vi "Weird Master.vi"() -> ()   [LabVIEW 2021]
uses:
  Transmission Data Unit/RTU/RTU Data Unit.lvclass
  API/Master/Modbus Master.lvclass
  Transmission Data Unit/ASCII/ASCII Data Unit.lvclass
  Network Protocol/Network Master/TCP/TCP Master.lvclass
  Master Function Definition/Master Function Definition.lvclass
  Transmission Data Unit/IP/IP Data Unit.lvclass
  Network Protocol/Network Master/Network Master.lvclass
  Transmission Data Unit/Transmission Data Unit.lvclass
  D:/my_projects/projects/Algorithms/Labview/21/Modbus_v121c/Transmission Data Unit/Transmission Data Unit.lvclass
  D:/my_projects/projects/Algorithms/Labview/21/Modbus_v121c/Transmission Data Unit/IP/IP Data Unit.lvclass
  D:/my_projects/projects/Algorithms/Labview/21/Modbus_v121c/Network Protocol/Network Master/Network Master.lvclass
  D:/my_projects/projects/Algorithms/Labview/21/Modbus_v121c/Network Protocol/Network Protocol.lvclass
  D:/my_projects/projects/Algorithms/Labview/21/Modbus_v121c/Network Protocol/Network Master/TCP/TCP Master.lvclass
  D:/my_projects/projects/Algorithms/Labview/21/Modbus_v121c/Transmission Data Unit/Serial Interface/Serial Data Unit.lvclass
  D:/my_projects/projects/Algorithms/Labview/21/Modbus_v121c/Transmission Data Unit/RTU/RTU Data Unit.lvclass
  D:/my_projects/projects/Algorithms/Labview/21/Modbus_v121c/Transmission Data Unit/ASCII/ASCII Data Unit.lvclass
  D:/my_projects/projects/Algorithms/Labview/21/Modbus_v121c/API/Modbus API.lvclass
  D:/my_projects/projects/Algorithms/Labview/21/Modbus_v121c/API/Master/Modbus Master.lvclass
  Data Model/Identification Parameters.ctl
  Data Model/Device Data Model.lvclass
  Master Function Definition/Read Device ID code.ctl
panel:
  in  "Serial Type":enum16{"RTU", "ASCII"}(ring)
  in  "Unit ID":u8=1
  out "loop time":dbl
  in  "Read Device ID code":T1
  in  "Object ID":u8
  out "Objects":T2[](array[typedef]) {"Object ID" format="%x"}
  out "exception status":u8
  out "discrete inputs":bool[](array[boolean])
  out "Input Registers":u16[](array[numeric])=[0, 0, 2, 2]
  out "error out":errorcluster
  out "Holding Registers":u16[](array[numeric])=[0, 0, 2, 2]
  in  "Write Single Register":u16[](array[numeric])=[0, 0, 2, 2]
  in  "Write Multiple Registers":cluster{"Set Registers":bool, u16[]}={"Set Registers"=FALSE, [0, 0, 2, 2]}
  in  "Write Multiple Coils":T3={"Write Single Coils 2"=[TRUE, FALSE, FALSE, TRUE], "Set Coils"=FALSE}
  in  "Write Single Coils":bool[](array[boolean])=[FALSE, FALSE, FALSE, FALSE] caption="Coils to Write"
  in  "Address":string="localhost"
  in  "Stop":bool
  out "Coils":bool[](array[boolean])=[TRUE, FALSE, FALSE, TRUE] caption="Slave Discrete Inputs"
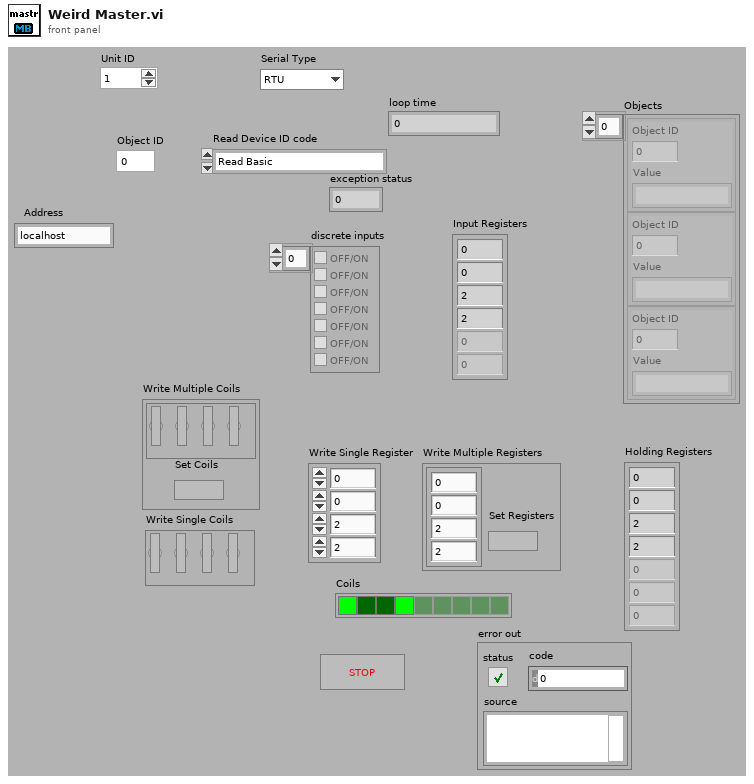
[diagram p1: front panel]
types:
  T1 = typedef "Device Data Model.lvclass/Read Device ID code.ctl" = enum8{"Read Basic", "Read Regular", "Read Extended", "Read Specific"}
  T2 = typedef "Device Data Model.lvclass/Identification Parameters.ctl" = cluster{"Object ID":u8, "Value":string}
  T3 = cluster{"Write Single Coils 2":bool[], "Set Coils":bool}
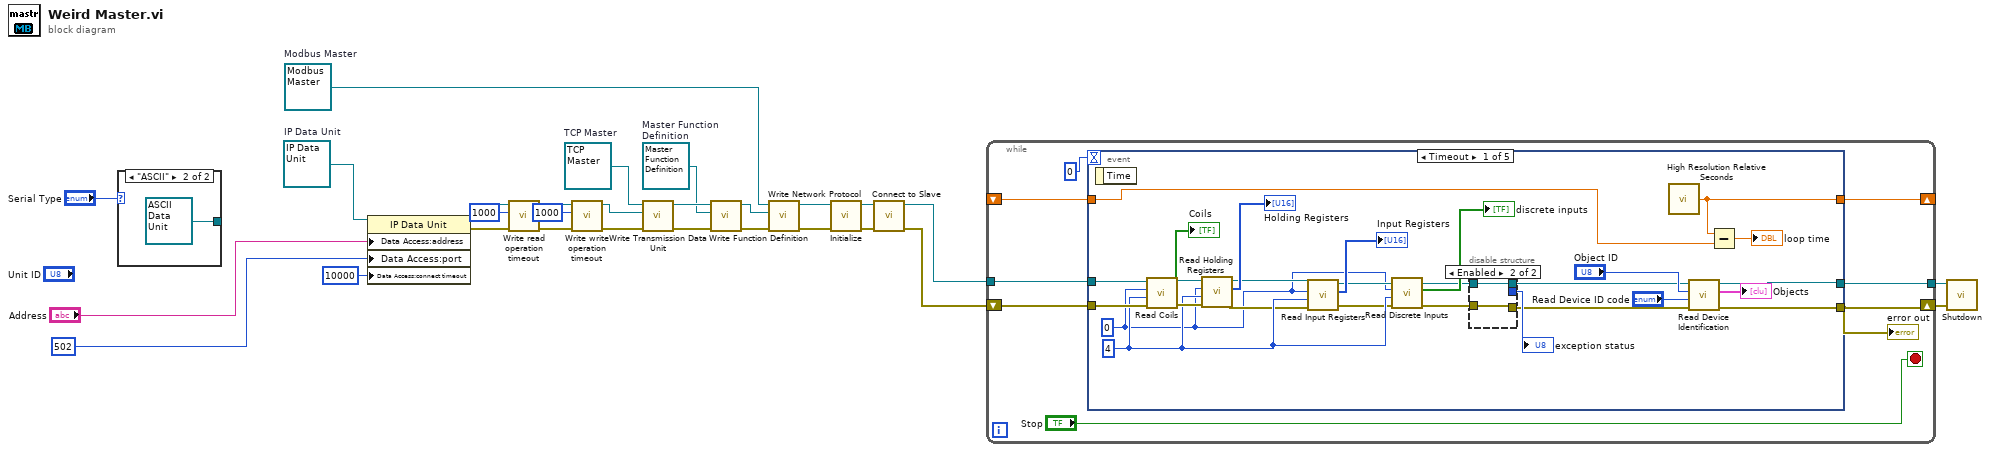
[diagram p0: block diagram]
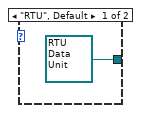
[diagram p2: hidden frame]
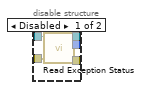
[diagram p3: hidden frame]
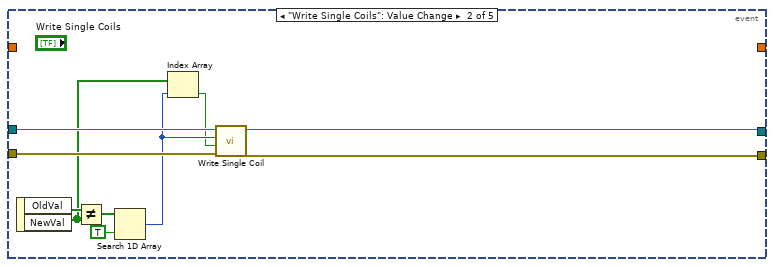
[diagram p4: hidden frame]
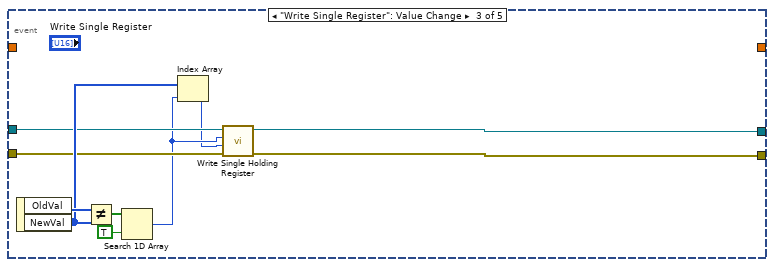
[diagram p5: hidden frame]
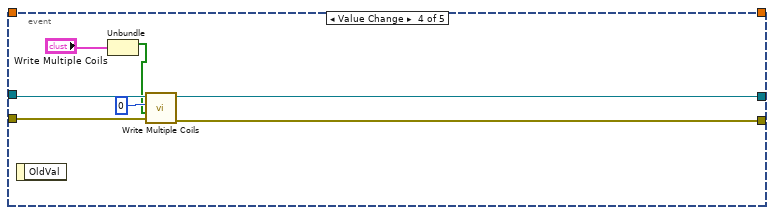
[diagram p6: hidden frame]
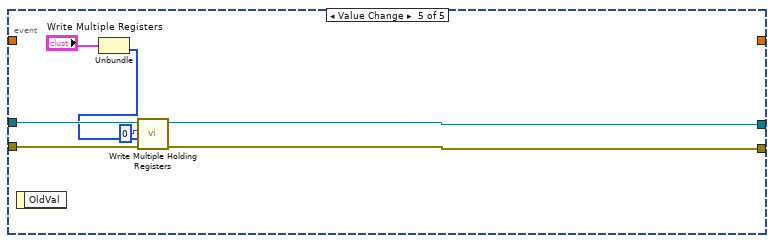
[diagram p7: hidden frame]
diagram:
  w19 = refnum<class "Modbus Master.lvclass"> refnum  # Modbus Master
  w21 = refnum<class "IP Data Unit.lvclass"> refnum  # IP Data Unit
  w10 = refnum<class "Master Function Definition.lvclass"> refnum  # Master Function Definition
  w20 = refnum<class "TCP Master.lvclass"> refnum  # TCP Master
  n1 = case shown="\"ASCII\"" "Serial Type" {
    tunnel: [refnum<class "RTU Data Unit.lvclass"> refnum ("RTU Data Unit") refnum<class "ASCII Data Unit.lvclass"> refnum ("ASCII Data Unit")] -> _
    frame "RTU", Default {
    }
    frame "ASCII" {
    }
  }
  n2 = property class="IP Data Unit"(reference=w21, "Data Access:address"="Address", "Data Access:port"=u16 502 ("Port"), "Data Access:connect timeout"=10000 ("connect timeout")) -> (reference out=w9:refnum<class "IP Data Unit.lvclass">, error out=w8:errorcluster)  [unwired: 1 in]
  n3 = call "Write read operation timeout.vi"("error in (no error)"=w8, "read operation timeout"=1000, "transmission data unit in"=w9) -> ("error out"=w22:errorcluster, "transmission data unit out"=w23:refnum<class "IP Data Unit.lvclass">)  [unwired: 7 in]
  n4 = call "Write write operation timeout.vi"("error in (no error)"=w22, "write operation timeout"=1000, "transmission data unit in"=w23) -> ("error out"=w18:errorcluster, "transmission data unit out"=w17:refnum<class "IP Data Unit.lvclass">)  [unwired: 7 in]
  n5 = call "Write Transmission Data Unit.vi"("error in (no error)"=w18, "Transmission Data Unit"=w17, "Network Master in"=w20) -> ("error out"=w12:errorcluster, "Network Master out"=w14:refnum<class "TCP Master.lvclass">)  [unwired: 7 in]
  n6 = call "Write Function Definition.vi"("error in"=w12, "master function definition"=w10, "Modbus master in"=w14) -> ("error out"=w11:errorcluster, "Modbus master out"=w13:refnum<class "TCP Master.lvclass">)  [unwired: 7 in]
  n7 = call "Write Network Protocol.vi"("error in (no error)"=w11, "Network Protocol"=w13, "Modbus API in"=w19) -> ("error out"=w15:errorcluster, "Modbus API out"=w16:refnum<class "Modbus Master.lvclass">)  [unwired: 7 in]
  n8 = call-dynamic "Initialize.vi"("error in (no error)"=w15, "Modbus master in"=w16) -> ("error out"=w1:errorcluster, "Modbus master out"=w2:refnum<class "Modbus Master.lvclass">)  [unwired: 8 in]
  n9 = call-dynamic "Connect to Slave.vi"("error in (no error)"=w1, "Modbus master in"=w2) -> ("error out"=w24:errorcluster, "Modbus master out"=w25:refnum<class "Modbus Master.lvclass">)  [unwired: 8 in]
  n10 = while {
    tunnel: w25 -> [w35]
    tunnel: [w34] -> w27
    shift-right: [w37] -> w28
    shift-left: w24 -> [w33]
    shift-right: [w32] -> _
    shift-left: _ -> [w31]
    stop <- "Stop" stop-if-true
    n11 = event shown="[0] Timeout" {
      selector: _ -> [_ _ _ _ _]
      dyn-events: _ -> [_ _ _ _ _]
      timeout: 0 -> [_ _ _ _ _]
      tunnel: [w42 w80 w88 w95 w102] -> w37
      tunnel: w35 -> [w65 w82 w86 w98 w104]
      tunnel: [w44 w79 w87 w94 w103] -> w34
      tunnel: w33 -> [w64 w81 w85 w97 w105]
      tunnel: [w41 _ _ _ _] -> w32
      tunnel: w31 -> [w40 _ _ _ _]
      event Timeout {
        w58 = u16 4 ("Number of coils")
        w51 = u16 0 ("Starting Address")
        n12 = event-data() -> ()  [unwired: 2 out]
        n13 = call-dynamic "Read Coils.vi"("error in (no error)"=w64, "number of coils"=w58, "starting address"=w51, "Modbus master in"=w65) -> ("error out"=w61:errorcluster, "coil values"=→"Coils":bool[], "Modbus master out"=w62:refnum<class "Modbus Master.lvclass">)  [unwired: 5 in]
        n14 = call-dynamic "Read Holding Registers.vi"("error in (no error)"=w61, "number of holding registers"=w58, "starting address"=w51, "Modbus master in"=w62) -> ("error out"=w54:errorcluster, "register values"=→"Holding Registers":u16[], "Modbus master out"=w55:refnum<class "Modbus Master.lvclass">)  [unwired: 5 in]
        n15 = call-dynamic "Read Input Registers.vi"("error in (no error)"=w54, "number of input registers"=w58, "starting address"=w51, "Modbus master in"=w55) -> ("error out"=w52:errorcluster, "register values"=→"Input Registers":u16[], "Modbus master out"=w53:refnum<class "Modbus Master.lvclass">)  [unwired: 5 in]
        n16 = call-dynamic "Read Discrete Inputs.vi"("error in (no error)"=w52, "number of discrete inputs"=w58, "starting address"=w51, "Modbus master in"=w53) -> ("error out"=w49:errorcluster, "discrete input values"=→"discrete inputs":bool[], "Modbus master out"=w50:refnum<class "Modbus Master.lvclass">)  [unwired: 5 in]
        n17 = disable-structure shown="Enabled" {
          disable-tunnel: [w70 _] -> w56
          disable-tunnel: w50 -> [w69 w71]
          disable-tunnel: w49 -> [w68 w72]
          disable-tunnel: [w67 w71] -> w45
          disable-tunnel: [w66 w72] -> w43
          frame Disabled {
            n18 = call-dynamic "Read Exception Status.vi"("error in (no error)"=w68, "Modbus master in"=w69) -> ("error out"=w66:errorcluster, "exception status"=w70:u8, "Modbus master out"=w67:refnum<class "Modbus Master.lvclass">)  [unwired: 7 in]
          }
          frame Enabled {
          }
        }
        "exception status" <- w56
        n19 = call <vilib>:"High Resolution Relative Seconds.vi"() -> ("relative seconds"=w41:dbl)
        n20 = call-dynamic "Read Device Identification.vi"("error in (no error)"=w43, "read device ID code"="Read Device ID code", "object ID"="Object ID", "Modbus master in"=w45) -> ("error out"=w42:errorcluster, "objects"=→"Objects":cluster{"object ID":u8, "value":string}[], "Modbus master out"=w44:refnum<class "Modbus Master.lvclass">)  [unwired: 5 in]
        n21 = Subtract(x=w41, y=w40) -> (x-y=→"loop time":dbl)
      }
      event "Write Single Coils": Value Change {
        n22 = event-data() -> ("OldVal"=w78:bool[], "NewVal"=w75:bool[])  [unwired: 1 out]
        n23 = Not Equal?(x=w78, y=w75) -> (x != y?=w77:bool[])
        n24 = Search 1D Array(1D array=w77, element=TRUE) -> (index of element=w74:i32)  [unwired: 1 in]
        n25 = Index Array(array=w75, index=w74) -> (element=w73:bool)
        n26 = call-dynamic "Write Single Coil.vi"("error in (no error)"=w81, "coil value"=w73, "address"=w74, "Modbus master in"=w82) -> ("error out"=w80:errorcluster, "Modbus master out"=w79:refnum<class "Modbus Master.lvclass">)  [unwired: 6 in]
      }
      event "Write Single Register": Value Change {
        n27 = event-data() -> ("OldVal"=w90:u16[], "NewVal"=w89:u16[])  [unwired: 1 out]
        n28 = Not Equal?(x=w90, y=w89) -> (x != y?=w92:bool[])
        n29 = Search 1D Array(1D array=w92, element=TRUE) -> (index of element=w84:i32)  [unwired: 1 in]
        n30 = Index Array(array=w89, index=w84) -> (element=w83:u16)
        n31 = call-dynamic "Write Single Holding Register.vi"("error in (no error)"=w85, "holding register value"=w83, "address"=w84, "Modbus master in"=w86) -> ("error out"=w88:errorcluster, "Modbus master out"=w87:refnum<class "Modbus Master.lvclass">)  [unwired: 6 in]
      }
      event "Write Multiple Coils.Set Coils": Value Change {
        n32 = event-data() -> ()  [unwired: 2 out]
        n33 = Unbundle("Write Multiple Coils") -> ("Write Single Coils 2"=w93:bool[])  [unwired: 1 out]
        n34 = call-dynamic "Write Multiple Coils.vi"("error in (no error)"=w97, "coil values"=w93, "starting address"=u16 0 ("Starting Address"), "Modbus master in"=w98) -> ("error out"=w95:errorcluster, "Modbus master out"=w94:refnum<class "Modbus Master.lvclass">)  [unwired: 6 in]
      }
      event "Write Multiple Registers.Set Registers": Value Change {
        n35 = event-data() -> ()  [unwired: 2 out]
        n36 = Unbundle("Write Multiple Registers") -> (w100:u16[])  [unwired: 1 out]
        n37 = call-dynamic "Write Multiple Holding Registers.vi"("error in (no error)"=w105, "holding register values"=w100, "starting address"=u16 0 ("Starting Address"), "Modbus master in"=w104) -> ("error out"=w102:errorcluster, "Modbus master out"=w103:refnum<class "Modbus Master.lvclass">)  [unwired: 6 in]
      }
    }
    "error out" <- w37
  }
  n38 = call-dynamic "Shutdown.vi"("error in (no error)"=w28, "Modbus master in"=w27) -> ()  [unwired: 9 in, 1 out]
